vi "Set Data (str) (子VI).vi"(8 "元素":T1={"initialize"="", "6221"={"6221 Resource"="GPIB0::24::INSTR", "Delta status"=FALSE}, "7001"={"Ch"=FALSE}, "SR830+6221"={"source"=0, "阻抗"=0.0, "量程入 4"=0, "量程入 3"=0, "量程入 2"=0, "量程入 1"=0, "电流"=0.0, "SR830 2"=FALSE, "SR830 3"=FALSE, "SR830 4"=FALSE, "SR830 1"=FALSE, "VISA 1"="", "VISA 2"="", "VISA 3"="", "VISA 4"="", "量程"=enum."量程每次测量会判定"}, "2400"={"2400"=FALSE, "VISA"=""}, "ch"={"ch str"="", "ch1"=FALSE, "ch2"=FALSE, "布尔"=FALSE}, "error"=FALSE, "数据文件路径"=path "", "log"={"log路径"=path "", "log interval"=0.0}, "Instrument"={"335 Resource"="GPIB0::24::INSTR", "Input (0:A)"=0, "Instrument Type"=3, "quantum design"=refnum, "Heater Output (1:1)"=1, "335state"=refnum, "semaphore"=refnum, "TCP master instance"=refnum}} {"Instrument"."Input (0:A)" items=["A", "B"]; "Instrument"."Instrument Type" items=["PPMS", "VersaLab", "DynaCool", "SVSM", "Lakeshore335", "PPMS-Rotate"]; "Instrument"."Heater Output (1:1)" items=["1"=1, "2"=2]; "SR830+6221"."source" items=["SR830 1", "SR830 2", "SR830 3", "SR830 4"]}, 11 "字符串":string) -> (0 "错误输出":errorcluster, 3 "path":path)   [LabVIEW 2019, in "Take Seq.lvlib"]
uses:
  Take Seq.lvlib
  config.ctl
  <vilib>/NI/Modbus Library/API/Master/Modbus Master.lvclass
  Instrument.ctl
  lib/QDInstrument.dll
panel:
  # "(真是通道1，假是通道2)"
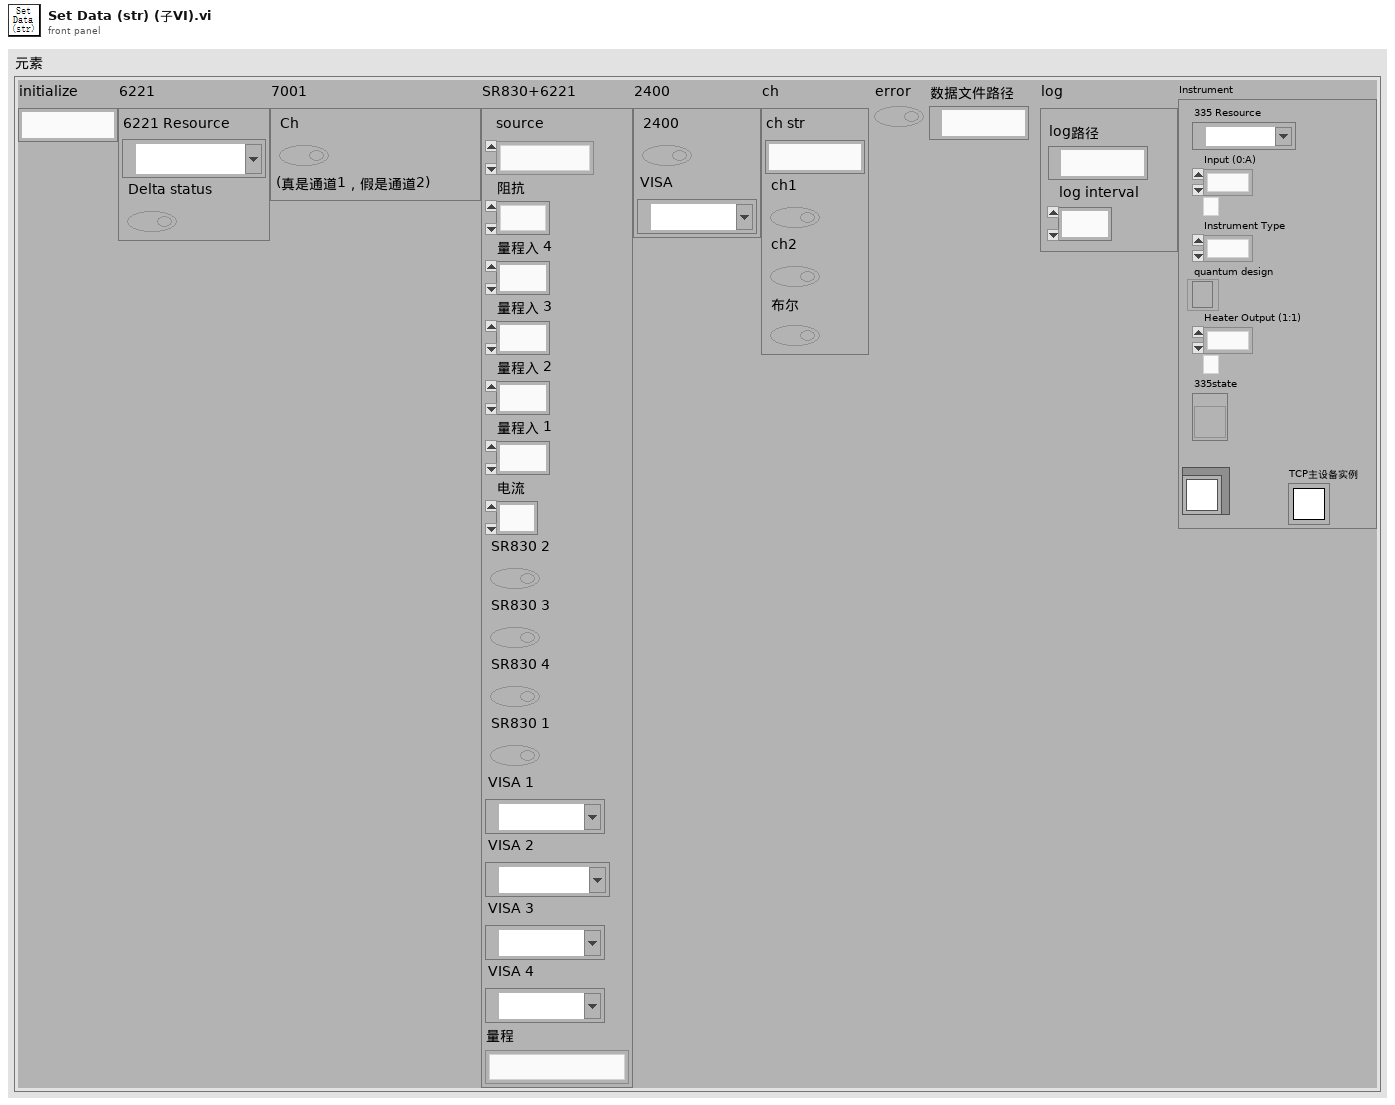
[diagram p1: front panel]
types:
  T1 = typedef "config.ctl" = cluster{"initialize":string, "6221":cluster{"6221 Resource":refnum<visa-resource-name>, "Delta status":bool}, "7001":cluster{"Ch":bool}, "SR830+6221":cluster{"source":u16, "阻抗":dbl, "量程入 4":i32, "量程入 3":i32, "量程入 2":i32, "量程入 1":i32, "电流":dbl, "SR830 2":bool, "SR830 3":bool, "SR830 4":bool, "SR830 1":bool, "VISA 1":refnum<visa-resource-name>, "VISA 2":refnum<visa-resource-name>, "VISA 3":refnum<visa-resource-name>, "VISA 4":refnum<visa-resource-name>, "量程":enum16{"量程每次测量会判定", "量程不变为设定值"}}, "2400":cluster{"2400":bool, "VISA":refnum<visa-resource-name>}, "ch":cluster{"ch str":string, "ch1":bool, "ch2":bool, "布尔":bool}, "error":bool, "数据文件路径":path, "log":cluster{"log路径":path, "log interval":dbl}, "Instrument":T2}
  T2 = typedef "Instrument.ctl" = cluster{"335 Resource":refnum<visa-resource-name>, "Input (0:A)":u16, "Instrument Type":i32, "quantum design":refnum<k24>, "Heater Output (1:1)":u16, "335state":refnum<vi>, "semaphore":T3, "TCP master instance":refnum<class "Modbus Master.lvclass">}
  T3 = typedef "Semaphore RefNum" = refnum<k1>
  T4 = enum16{"open", "replace", "create", "open or create", "replace or create", "replace or create with confirmation"}
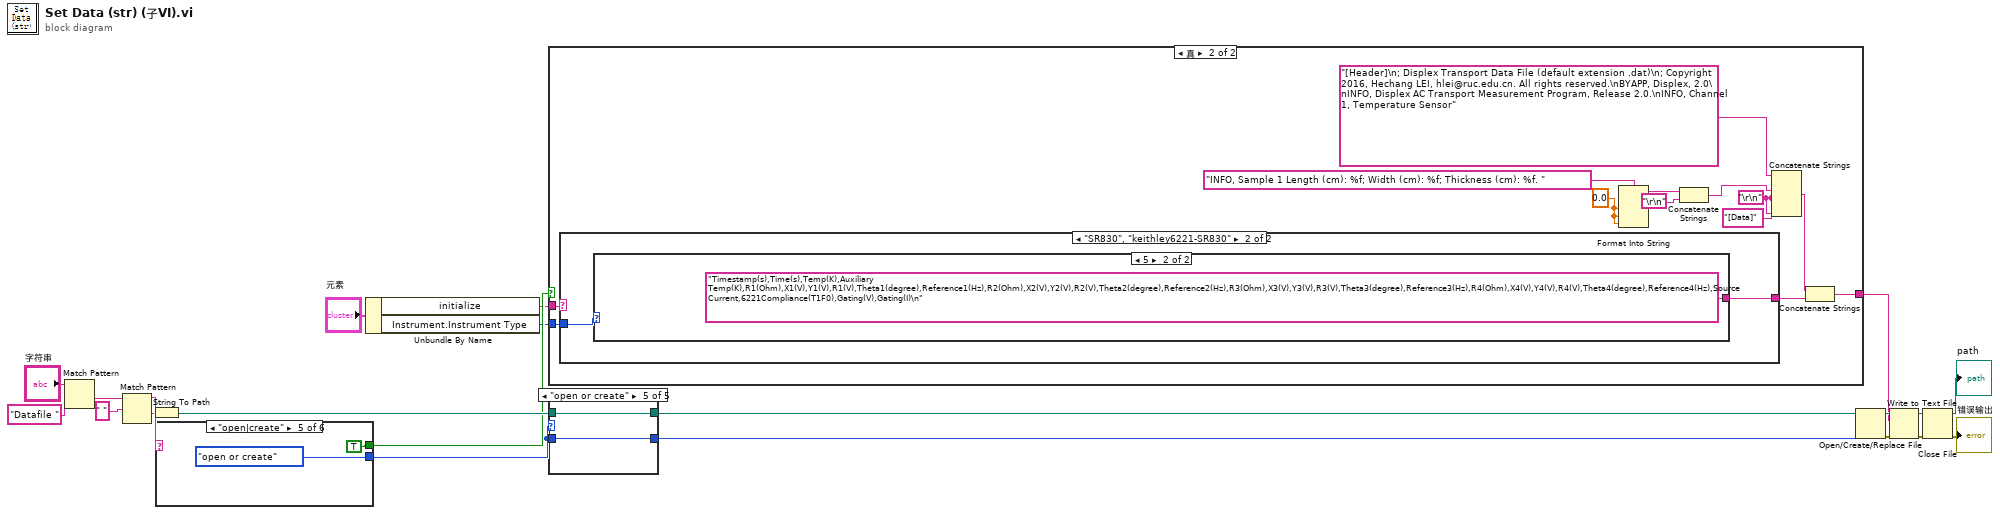
[diagram p0: block diagram]
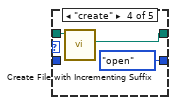
[diagram p5: hidden frame]
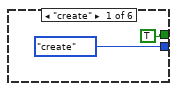
[diagram p6: hidden frame]
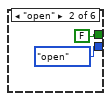
[diagram p7: hidden frame]
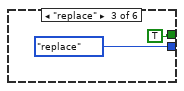
[diagram p8: hidden frame]
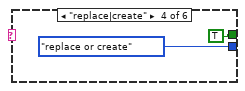
[diagram p9: hidden frame]
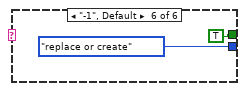
[diagram p10: hidden frame]
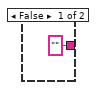
[diagram p11: hidden frame]
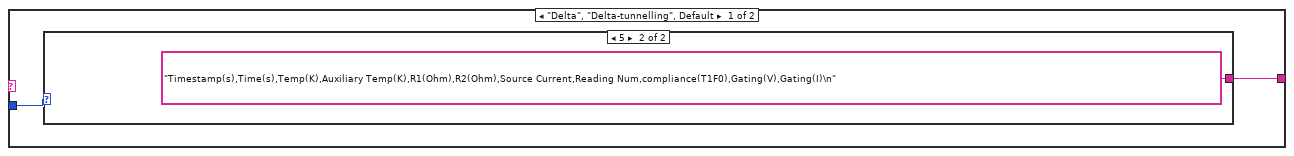
[diagram p12: hidden frame]
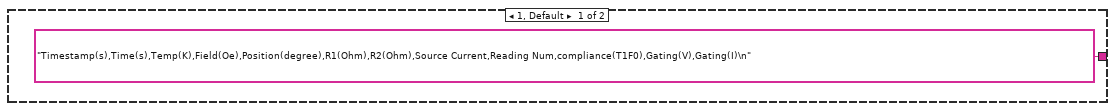
[diagram p13: hidden frame]
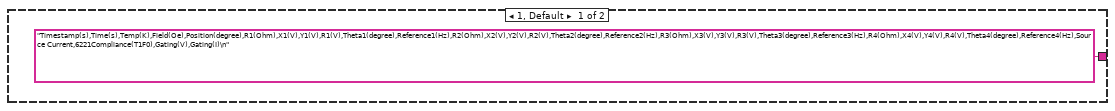
[diagram p14: hidden frame]
diagram:
  n1 = Match Pattern(string="字符串", regular expression="Datafile " ("正则表达式")) -> (after substring=w8:string)  [unwired: 1 in, 3 out]
  n2 = Match Pattern(string=w8, regular expression=" " ("正则表达式")) -> (before substring=w20:string, after substring=w10:string)  [unwired: 1 in, 2 out]
  n3 = String To Path(string=w10) -> (path=w16:path)
  n4 = case shown="\"open|create\"" w20 {
    tunnel: [T4."create" ("操作(0:open)") T4."open" ("操作(0:open)") T4."replace" ("操作(0:open)") T4."replace or create" ("操作(0:open)") T4."open or create" ("操作(0:open)") T4."replace or create" ("操作(0:open)")] -> w18
    tunnel: [TRUE FALSE TRUE TRUE TRUE TRUE] -> w11
    frame "create" {
    }
    frame "open" {
    }
    frame "replace" {
    }
    frame "replace|create" {
    }
    frame "open|create" {
    }
    frame "-1", Default {
    }
  }
  n5 = Unbundle By Name("元素") -> ("initialize"=w2:string, "Instrument.Instrument Type"=w1:i32)
  n6 = case shown="真" w11 {
    tunnel: ["" w36] -> w5
    tunnel: w2 -> [_ w47]
    tunnel: w1 -> [_ w35]
    frame False {
    }
    frame True {
      w43 = 0.0 ("输入 1")
      w40 = "\r\n"
      n7 = case shown="\"SR830\", \"keithley6221-SR830\"" w47 {
        tunnel: [w49 w53] -> w37
        tunnel: w35 -> [w48 w52]
        frame "Delta", "Delta-tunnelling", Default {
          n8 = case shown="5" w48 {
            tunnel: ["Timestamp(s),Time(s),Temp(K),Field(Oe),Position(degree),R1(Ohm),R2(Ohm),Source Current,Reading Num,compliance(T1F0),Gating(V),Gating(I)\n" ("字符串") "Timestamp(s),Time(s),Temp(K),Auxiliary Temp(K),R1(Ohm),R2(Ohm),Source Current,Reading Num,compliance(T1F0),Gating(V),Gating(I)\n" ("字符串")] -> w49
            frame 1, Default {
            }
            frame 5 {
            }
          }
        }
        frame "SR830", "keithley6221-SR830" {
          n9 = case shown="5" w52 {
            tunnel: ["Timestamp(s),Time(s),Temp(K),Field(Oe),Position(degree),R1(Ohm),X1(V),Y1(V),R1(V),Theta1(degree),Reference1(Hz),R2(Ohm),X2(V),Y2(V),R2(V),Theta2(degree),Reference2(Hz),R3(Ohm),X3(V),Y3(V),R3(V),Theta3(degree),Reference3(Hz),R4(Ohm),X4(V),Y4(V),R4(V),Theta4(degree),Reference4(Hz),Source Current,6221Compliance(T1F0),Gating(V),Gating(I)\n" ("字符串") "Timestamp(s),Time(s),Temp(K),Auxiliary Temp(K),R1(Ohm),X1(V),Y1(V),R1(V),Theta1(degree),Reference1(Hz),R2(Ohm),X2(V),Y2(V),R2(V),Theta2(degree),Reference2(Hz),R3(Ohm),X3(V),Y3(V),R3(V),Theta3(degree),Reference3(Hz),R4(Ohm),X4(V),Y4(V),R4(V),Theta4(degree),Reference4(Hz),Source Current,6221Compliance(T1F0),Gating(V),Gating(I)\n" ("字符串")] -> w53
            frame 1, Default {
            }
            frame 5 {
            }
          }
        }
      }
      n10 = Format Into String(format string="INFO, Sample 1 Length (cm): %f; Width (cm): %f; Thickness (cm): %f. " ("string"), w43, w43, w43) -> (resulting string=w46:string)  [unwired: 2 in, 1 out]
      n11 = Concatenate Strings(w46, "\r\n") -> (w45:string)
      n12 = Concatenate Strings("[Header]\n; Displex Transport Data File (default extension .dat)\n; Copyright 2016, Hechang LEI, hlei@ruc.edu.cn. All rights reserved.\nBYAPP, Displex, 2.0\nINFO, Displex AC Transport Measurement Program, Release 2.0.\nINFO, Channel 1, Temperature Sensor" ("string"), w40, w45, w40, "[Data]" ("string"), w40) -> (w38:string)
      n13 = Concatenate Strings(w38, w37) -> (w36:string)
    }
  }
  n14 = case shown="\"open or create\"" w18 {
    tunnel: w16 -> [w57 w59 w61 w64 w66]
    tunnel: [w57 w59 w61 w63 w66] -> w17
    tunnel: [w56 w58 w60 T4."open" ("操作(0:open)") w65] -> w19
    tunnel: w18 -> [w56 w58 w60 _ w65]
    frame "open", Default {
    }
    frame "replace" {
    }
    frame "replace or create" {
    }
    frame "create" {
      n15 = call <vilib>:"Create File with Incrementing Suffix.vi"("file path"=w64) -> ("actual path"=w63:path)  [unwired: 8 in, 2 out]
    }
    frame "open or create" {
    }
  }
  n16 = Open/Create/Replace File(file path (use dialog)=w17, operation (0:open)=w19) -> (refnum out=w12:refnum<file>, error out=w14:errorcluster)  [unwired: 4 in, 1 out]
  n17 = Write to Text File(file (use dialog)=w12, text=w5, error in=w14) -> (refnum out=w21:refnum<file>, error out=w4:errorcluster)  [unwired: 1 in, 1 out]
  n18 = Close File(refnum=w21, error in=w4) -> (path=→"path":path, error out=→"错误输出":errorcluster)
